vi "Integral.vi"(8 "error in (no error)":errorcluster, 11 "PID in":refnum<class "PID.lvclass">) -> (0 "error out":errorcluster, 3 "PID out":refnum<class "PID.lvclass">)   [LabVIEW 2025, in "PID.lvlib" / "PID.lvclass"]
uses:
  PID.lvclass
  PID.lvclass/PID.ctl
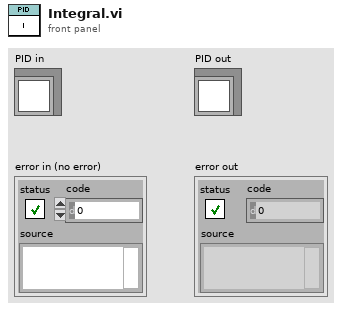
[diagram p1: front panel]
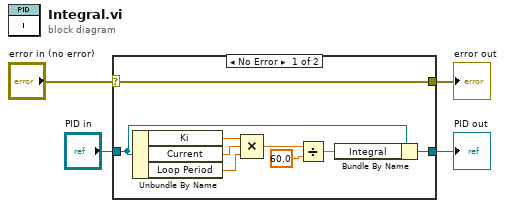
[diagram p0: block diagram]
diagram:
  n1 = case shown="No Error" "error in (no error)" {
    selector: "error in (no error)" -> [w5 w15]
    tunnel: [w5 w15] -> w3
    tunnel: [w8 w14] -> w1
    tunnel: "PID in" -> [w7 w14]
    frame No Error {
      n2 = Unbundle By Name(w7) -> ("Ki"=w13:dbl, "Current"=w6:dbl, "Loop Period"=w12:dbl)
      n3 = Compound Arithmetic op=MULTIPLY(w13, w6, w12) -> (w11:dbl)
      n4 = Divide(x=w11, y=60.0) -> (x/y=w9:dbl)
      n5 = Bundle By Name(cluster=w7, "Integral"=w9) -> (w8:refnum<class "PID.lvclass">)
    }
    frame Error {
    }
  }
  "error out" <- w3
  "PID out" <- w1
